vi "intensity_function.vi"(6 "theta_min":dbl, 8 "theta":dbl, 9 "C":dbl, 10 "B":dbl, 11 "A":dbl) -> (3 "output variable":dbl)   [LabVIEW 2019]
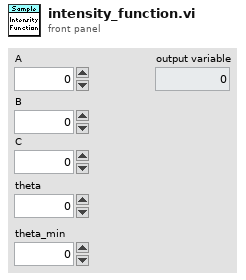
[diagram p1: front panel]
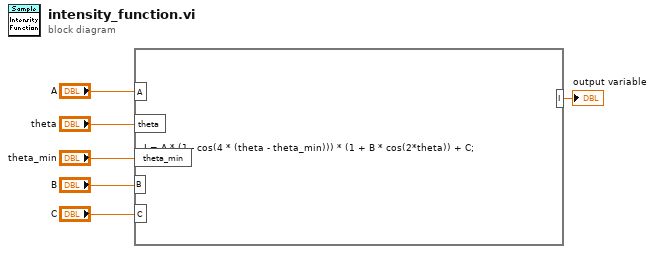
[diagram p0: block diagram]
diagram:
  n1 = formula code="I = A * (1 - cos(4 * (theta - theta_min))) * (1 + B * cos(2*theta)) + C;"("A"="A", "theta"="theta", "theta_min"="theta_min", "B"="B", "C"="C") -> ("I"=→"output variable":dbl)
